vi "Set64PinPGA.vi"(11 "Pattern":T2) -> (3 "64-Pin PGA":T1)   [LabVIEW 2012, in "Virtual-PGA.lvlib"]
uses:
  Virtual-PGA.lvlib
  Controls/Pattern.ctl
  Controls/Input.ctl
  Controls/64PinPGASmall.ctl
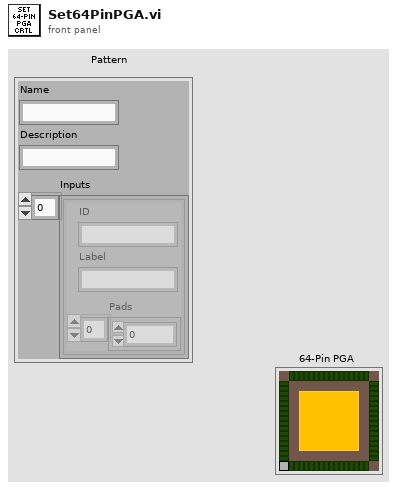
[diagram p1: front panel]
types:
  T1 = typedef "Virtual-PGA.lvlib/64PinPGASmall.ctl" = cluster{"Pad 49":bool, "Pad 50":bool, "Pad 51":bool, "Pad 52":bool, "Pad 53":bool, "Pad 54":bool, "Pad 55":bool, "Pad 56":bool, "Pad 57":bool, "Pad 58":bool, "Pad 59":bool, "Pad 60":bool, "Pad 61":bool, "Pad 62":bool, "Pad 63":bool, "Pad 64":bool, "Pad 32":bool, "Pad 31":bool, "Pad 30":bool, "Pad 29":bool, "Pad 28":bool, "Pad 27":bool, "Pad 26":bool, "Pad 25":bool, "Pad 24":bool, "Pad 23":bool, "Pad 22":bool, "Pad 21":bool, "Pad 20":bool, "Pad 19":bool, "Pad 18":bool, "Pad 17":bool, "Pad 1":bool, "Pad 2":bool, "Pad 3":bool, "Pad 4":bool, "Pad 5":bool, "Pad 6":bool, "Pad 7":bool, "Pad 8":bool, "Pad 9":bool, "Pad 10":bool, "Pad 11":bool, "Pad 12":bool, "Pad 13":bool, "Pad 14":bool, "Pad 15":bool, "Pad 16":bool, "Pad 48":bool, "Pad 47":bool, "Pad 46":bool, "Pad 45":bool, "Pad 44":bool, "Pad 43":bool, "Pad 42":bool, "Pad 41":bool, "Pad 40":bool, "Pad 39":bool, "Pad 38":bool, "Pad 37":bool, "Pad 36":bool, "Pad 35":bool, "Pad 34":bool, "Pad 33":bool}
  T2 = typedef "Virtual-PGA.lvlib/Pattern.ctl" = cluster{"Name":string, "Description":string, "Inputs":T3[]}
  T3 = typedef "Virtual-PGA.lvlib/Input.ctl" = cluster{"ID":string, "Label":string, "Pads":u32[]}
  T4 = cluster{"Y1":bool, "Y2":bool, "Y3":bool, "Y4":bool}[]
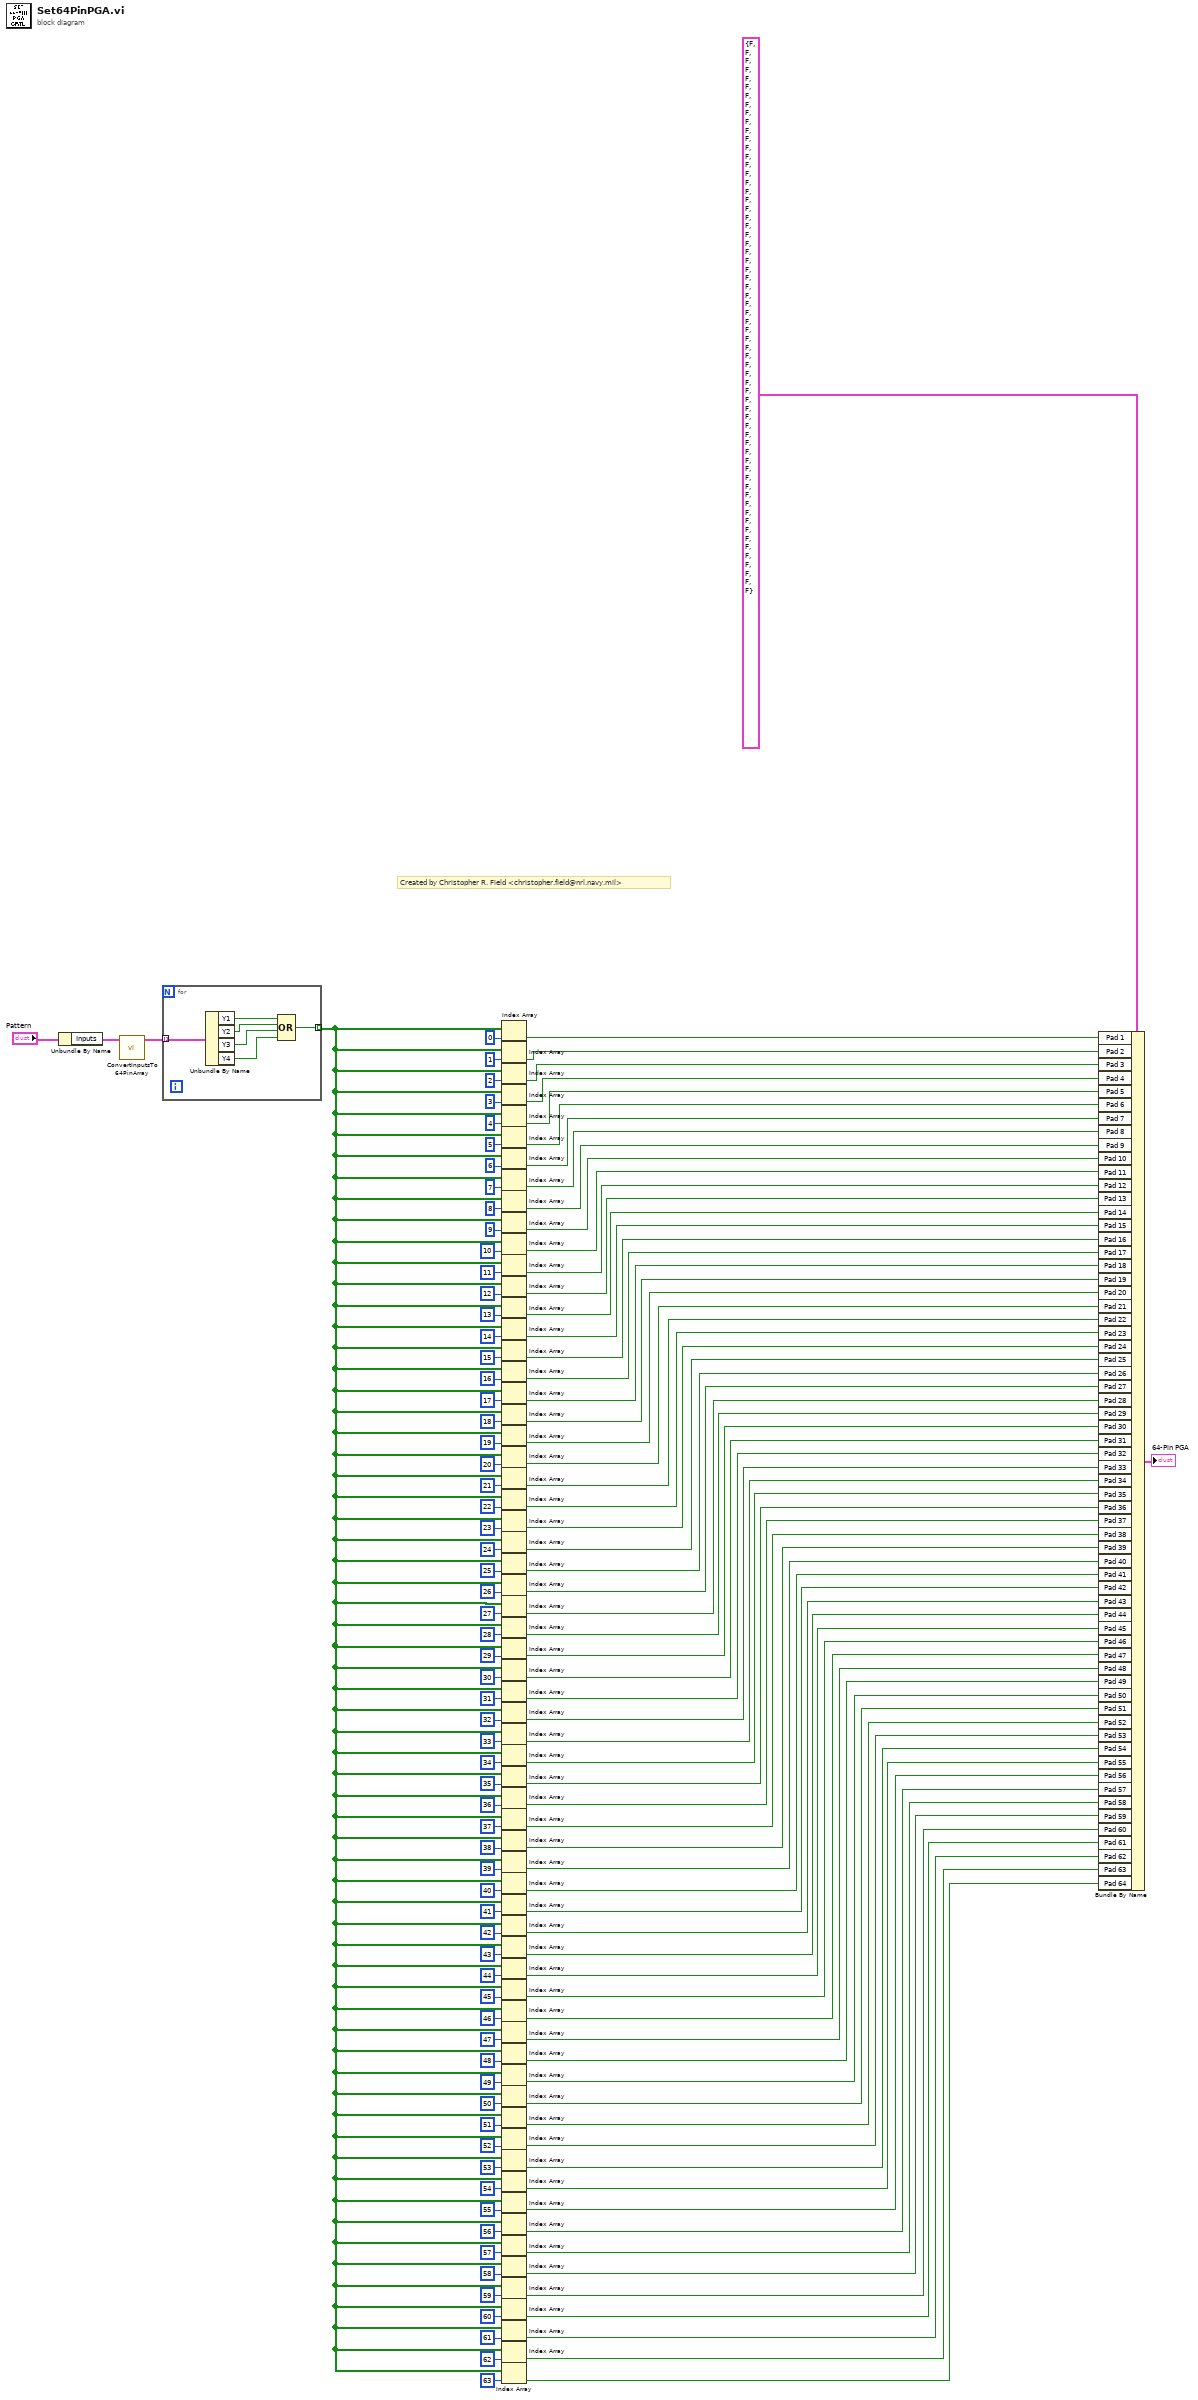
[diagram p0: block diagram]
diagram:
  # "Created by Christopher R. Field <christopher.field@nrl.navy.mil>"
  n1 = Unbundle By Name("Pattern") -> ("Inputs"=w8:T3[])
  n2 = call "ConvertInputsTo64PinArray.vi"("Inputs"=w8) -> ("64-Pin Array"=w7:T4)  [unwired: 10 in]
  n3 = for {
    tunnel: [w136] -> w4 mode=indexing
    tunnel: w7 -> [w135] mode=indexing
    n4 = Unbundle By Name(w135) -> ("Y1"=w140:bool, "Y2"=w139:bool, "Y3"=w138:bool, "Y4"=w137:bool)
    n5 = Compound Arithmetic op=OR(w140, w139, w138, w137) -> (w136:bool)
  }
  n6 = Index Array(array=w4, index=0) -> (element=w133:bool)
  n7 = Index Array(array=w4, index=1) -> (element=w131:bool)
  n8 = Index Array(array=w4, index=2) -> (element=w129:bool)
  n9 = Index Array(array=w4, index=3) -> (element=w2:bool)
  n10 = Index Array(array=w4, index=4) -> (element=w126:bool)
  n11 = Index Array(array=w4, index=5) -> (element=w124:bool)
  n12 = Index Array(array=w4, index=6) -> (element=w122:bool)
  n13 = Index Array(array=w4, index=7) -> (element=w64:bool)
  n14 = Index Array(array=w4, index=8) -> (element=w63:bool)
  n15 = Index Array(array=w4, index=9) -> (element=w62:bool)
  n16 = Index Array(array=w4, index=10) -> (element=w61:bool)
  n17 = Index Array(array=w4, index=11) -> (element=w60:bool)
  n18 = Index Array(array=w4, index=12) -> (element=w59:bool)
  n19 = Index Array(array=w4, index=13) -> (element=w58:bool)
  n20 = Index Array(array=w4, index=14) -> (element=w57:bool)
  n21 = Index Array(array=w4, index=15) -> (element=w56:bool)
  n22 = Index Array(array=w4, index=16) -> (element=w55:bool)
  n23 = Index Array(array=w4, index=17) -> (element=w54:bool)
  n24 = Index Array(array=w4, index=18) -> (element=w53:bool)
  n25 = Index Array(array=w4, index=19) -> (element=w52:bool)
  n26 = Index Array(array=w4, index=20) -> (element=w51:bool)
  n27 = Index Array(array=w4, index=21) -> (element=w50:bool)
  n28 = Index Array(array=w4, index=22) -> (element=w49:bool)
  n29 = Index Array(array=w4, index=23) -> (element=w48:bool)
  n30 = Index Array(array=w4, index=24) -> (element=w47:bool)
  n31 = Index Array(array=w4, index=25) -> (element=w46:bool)
  n32 = Index Array(array=w4, index=26) -> (element=w45:bool)
  n33 = Index Array(array=w4, index=27) -> (element=w44:bool)
  n34 = Index Array(array=w4, index=28) -> (element=w43:bool)
  n35 = Index Array(array=w4, index=29) -> (element=w42:bool)
  n36 = Index Array(array=w4, index=30) -> (element=w41:bool)
  n37 = Index Array(array=w4, index=31) -> (element=w40:bool)
  n38 = Index Array(array=w4, index=32) -> (element=w39:bool)
  n39 = Index Array(array=w4, index=33) -> (element=w38:bool)
  n40 = Index Array(array=w4, index=34) -> (element=w37:bool)
  n41 = Index Array(array=w4, index=35) -> (element=w36:bool)
  n42 = Index Array(array=w4, index=36) -> (element=w35:bool)
  n43 = Index Array(array=w4, index=37) -> (element=w34:bool)
  n44 = Index Array(array=w4, index=38) -> (element=w33:bool)
  n45 = Index Array(array=w4, index=39) -> (element=w32:bool)
  n46 = Index Array(array=w4, index=40) -> (element=w31:bool)
  n47 = Index Array(array=w4, index=41) -> (element=w30:bool)
  n48 = Index Array(array=w4, index=42) -> (element=w29:bool)
  n49 = Index Array(array=w4, index=43) -> (element=w28:bool)
  n50 = Index Array(array=w4, index=44) -> (element=w27:bool)
  n51 = Index Array(array=w4, index=45) -> (element=w26:bool)
  n52 = Index Array(array=w4, index=46) -> (element=w25:bool)
  n53 = Index Array(array=w4, index=47) -> (element=w24:bool)
  n54 = Index Array(array=w4, index=48) -> (element=w23:bool)
  n55 = Index Array(array=w4, index=49) -> (element=w5:bool)
  n56 = Index Array(array=w4, index=50) -> (element=w22:bool)
  n57 = Index Array(array=w4, index=51) -> (element=w21:bool)
  n58 = Index Array(array=w4, index=52) -> (element=w20:bool)
  n59 = Index Array(array=w4, index=53) -> (element=w19:bool)
  n60 = Index Array(array=w4, index=54) -> (element=w18:bool)
  n61 = Index Array(array=w4, index=55) -> (element=w17:bool)
  n62 = Index Array(array=w4, index=56) -> (element=w16:bool)
  n63 = Index Array(array=w4, index=57) -> (element=w15:bool)
  n64 = Index Array(array=w4, index=58) -> (element=w14:bool)
  n65 = Index Array(array=w4, index=59) -> (element=w13:bool)
  n66 = Index Array(array=w4, index=60) -> (element=w12:bool)
  n67 = Index Array(array=w4, index=61) -> (element=w11:bool)
  n68 = Index Array(array=w4, index=62) -> (element=w10:bool)
  n69 = Index Array(array=w4, index=63) -> (element=w6:bool)
  n70 = Bundle By Name(cluster=T1 {"Pad 49"=FALSE, "Pad 50"=FALSE, "Pad 51"=FALSE, "Pad 52"=FALSE, "Pad 53"=FALSE, "Pad 54"=FALSE, "Pad 55"=FALSE, "Pad 56"=FALSE, "Pad 57"=FALSE, "Pad 58"=FALSE, "Pad 59"=FALSE, "Pad 60"=FALSE, "Pad 61"=FALSE, "Pad 62"=FALSE, "Pad 63"=FALSE, "Pad 64"=FALSE, "Pad 32"=FALSE, "Pad 31"=FALSE, "Pad 30"=FALSE, "Pad 29"=FALSE, "Pad 28"=FALSE, "Pad 27"=FALSE, "Pad 26"=FALSE, "Pad 25"=FALSE, "Pad 24"=FALSE, "Pad 23"=FALSE, "Pad 22"=FALSE, "Pad 21"=FALSE, "Pad 20"=FALSE, "Pad 19"=FALSE, "Pad 18"=FALSE, "Pad 17"=FALSE, "Pad 1"=FALSE, "Pad 2"=FALSE, "Pad 3"=FALSE, "Pad 4"=FALSE, "Pad 5"=FALSE, "Pad 6"=FALSE, "Pad 7"=FALSE, "Pad 8"=FALSE, "Pad 9"=FALSE, "Pad 10"=FALSE, "Pad 11"=FALSE, "Pad 12"=FALSE, "Pad 13"=FALSE, "Pad 14"=FALSE, "Pad 15"=FALSE, "Pad 16"=FALSE, "Pad 48"=FALSE, "Pad 47"=FALSE, "Pad 46"=FALSE, "Pad 45"=FALSE, "Pad 44"=FALSE, "Pad 43"=FALSE, "Pad 42"=FALSE, "Pad 41"=FALSE, "Pad 40"=FALSE, "Pad 39"=FALSE, "Pad 38"=FALSE, "Pad 37"=FALSE, "Pad 36"=FALSE, "Pad 35"=FALSE, "Pad 34"=FALSE, "Pad 33"=FALSE} ("64-Pin PGA"), "Pad 1"=w133, "Pad 2"=w131, "Pad 3"=w129, "Pad 4"=w2, "Pad 5"=w126, "Pad 6"=w124, "Pad 7"=w122, "Pad 8"=w64, "Pad 9"=w63, "Pad 10"=w62, "Pad 11"=w61, "Pad 12"=w60, "Pad 13"=w59, "Pad 14"=w58, "Pad 15"=w57, "Pad 16"=w56, "Pad 17"=w55, "Pad 18"=w54, "Pad 19"=w53, "Pad 20"=w52, "Pad 21"=w51, "Pad 22"=w50, "Pad 23"=w49, "Pad 24"=w48, "Pad 25"=w47, "Pad 26"=w46, "Pad 27"=w45, "Pad 28"=w44, "Pad 29"=w43, "Pad 30"=w42, "Pad 31"=w41, "Pad 32"=w40, "Pad 33"=w39, "Pad 34"=w38, "Pad 35"=w37, "Pad 36"=w36, "Pad 37"=w35, "Pad 38"=w34, "Pad 39"=w33, "Pad 40"=w32, "Pad 41"=w31, "Pad 42"=w30, "Pad 43"=w29, "Pad 44"=w28, "Pad 45"=w27, "Pad 46"=w26, "Pad 47"=w25, "Pad 48"=w24, "Pad 49"=w23, "Pad 50"=w5, "Pad 51"=w22, "Pad 52"=w21, "Pad 53"=w20, "Pad 54"=w19, "Pad 55"=w18, "Pad 56"=w17, "Pad 57"=w16, "Pad 58"=w15, "Pad 59"=w14, "Pad 60"=w13, "Pad 61"=w12, "Pad 62"=w11, "Pad 63"=w10, "Pad 64"=w6) -> (→"64-Pin PGA":T1)
